vi "SUB wave2XY.vi"(1 "waveform":waveform(dbl)) -> (0 "output cluster":cluster{"xarray":dbl[], "yarray":dbl[]})   [LabVIEW 2017]
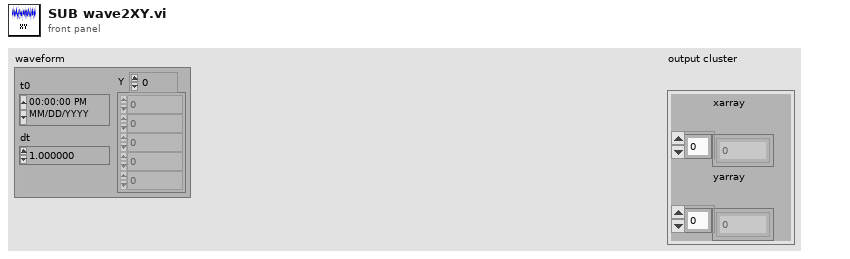
[diagram p1: front panel]
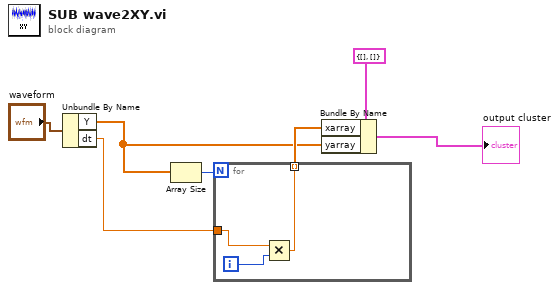
[diagram p0: block diagram]
diagram:
  n1 = Unbundle By Name("waveform") -> ("Y"=w2:dbl[], "dt"=w5:dbl)
  n2 = Array Size(array=w2) -> (size(s)=w6:i32)
  n3 = for {
    N: w6 -> [_]
    tunnel: w5 -> [w9]
    tunnel: [w8] -> w3 mode=indexing
    i -> [w10]
    n4 = Multiply(x=w9, y=w10) -> (x*y=w8:dbl)
  }
  n5 = Bundle By Name(cluster=cluster{"xarray":dbl[], "yarray":dbl[]} {"xarray"=[], "yarray"=[]} ("XYarray"), "xarray"=w3, "yarray"=w2) -> (→"output cluster":cluster{"xarray":dbl[], "yarray":dbl[]})
